vi "PCO_RecorderSaveOverlay_B8.vi"(0 "pImgBufR":u8[][](array[numeric])=array1x4097[4097 elements], 1 "pImgBufG":u8[][](array[numeric])=array1x4097[4097 elements], 2 "pImgBufB":u8[][](array[numeric])=array1x4097[4097 elements], 3 "wWidth":u16, 4 "wHeight":u16, 5 "error in (no error)":errorcluster {"code" format="%x"}, 8 "PCO_METADATA_STRUCT":T1, 9 "szFilePath":path, 11 "bOverwrite":bool) -> (14 "ErrorMessage":i32 format="%x", 19 "error out":errorcluster {"code" format="%x"})   [LabVIEW 2019, in "Recorder.lvlib"]
doc: "int WINAPI PCO_RecorderSaveOverlay(void* pImgBufR, void* pImgBufG, void* pImgBufB, WORD wWidth, WORD wHeight, const char* cFileType, const char* szFilePath, bool bOverwrite, PCO_METADATA_STRUCT* strMetadata);"
uses:
  Recorder.lvlib
  pco.sdk/Structures/Structures.lvlib
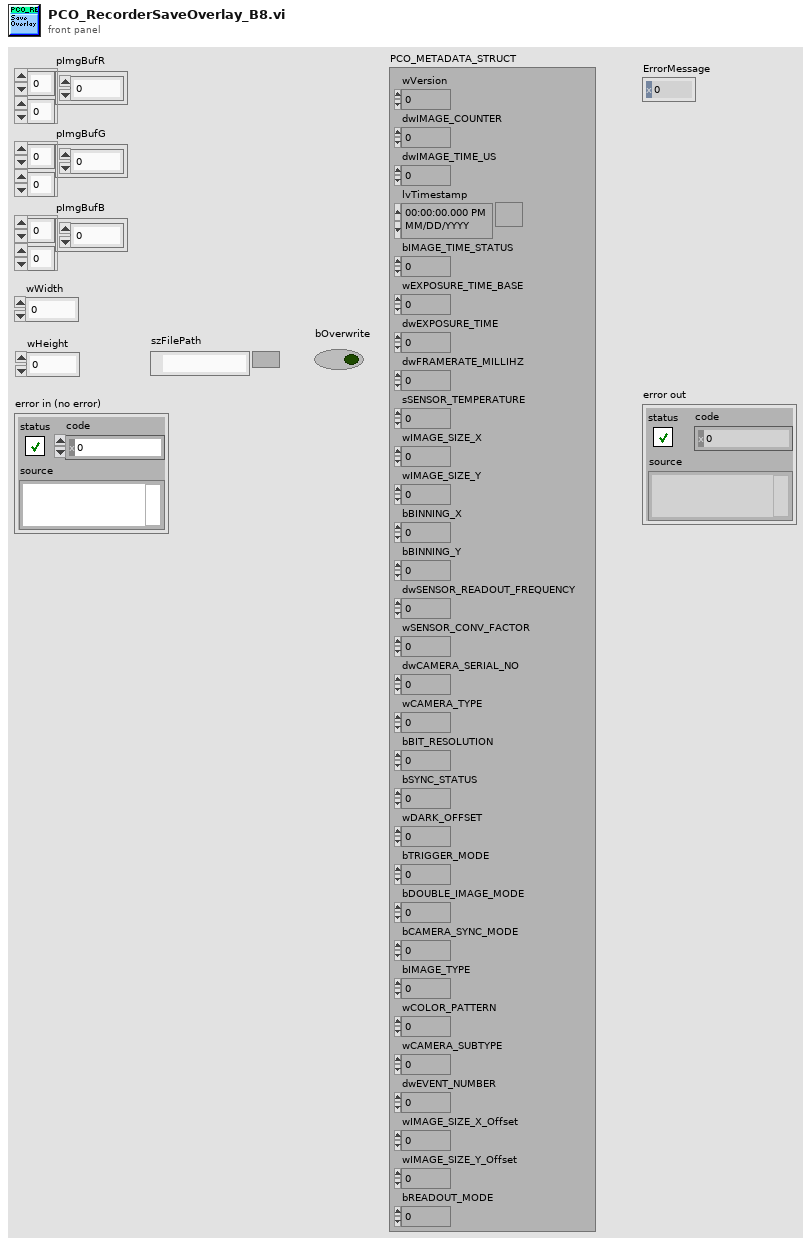
[diagram p1: front panel]
types:
  T1 = cluster{"wVersion":u16, "dwIMAGE_COUNTER":u32, "dwIMAGE_TIME_US":u32, "lvTimestamp":timestamp, "bIMAGE_TIME_STATUS":u8, "wEXPOSURE_TIME_BASE":u16, "dwEXPOSURE_TIME":u32, "dwFRAMERATE_MILLIHZ":u32, "sSENSOR_TEMPERATURE":i16, "wIMAGE_SIZE_X":u16, "wIMAGE_SIZE_Y":u16, "bBINNING_X":u8, "bBINNING_Y":u8, "dwSENSOR_READOUT_FREQUENCY":u32, "wSENSOR_CONV_FACTOR":u16, "dwCAMERA_SERIAL_NO":u32, "wCAMERA_TYPE":u16, "bBIT_RESOLUTION":u8, "bSYNC_STATUS":u8, "wDARK_OFFSET":u16, "bTRIGGER_MODE":u8, "bDOUBLE_IMAGE_MODE":u8, "bCAMERA_SYNC_MODE":u8, "bIMAGE_TYPE":u8, "wCOLOR_PATTERN":u16, "wCAMERA_SUBTYPE":u16, "dwEVENT_NUMBER":u32, "wIMAGE_SIZE_X_Offset":u16, "wIMAGE_SIZE_Y_Offset":u16, "bREADOUT_MODE":u8}
  T2 = typedef "LVDateTimeRec.ctl" = cluster{"fractional second":dbl, "second":i32, "minute":i32, "hour":i32, "day of month":i32, "month":i32, "year":i32, "day of week":i32, "day of year":i32, "DST":i32}
  T3 = cluster{"wSize":u16, "wVersion":u16, "bIMAGE_COUNTER_BCD":cluster{u8, u8, u8, u8}, "bIMAGE_TIME_US_BCD":cluster{u8, u8, u8}, "bIMAGE_TIME_SEC_BCD":u8, "bIMAGE_TIME_MIN_BCD":u8, "bIMAGE_TIME_HOUR_BCD":u8, "bIMAGE_TIME_DAY_BCD":u8, "bIMAGE_TIME_MON_BCD":u8, "bIMAGE_TIME_YEAR_BCD":u8, "bIMAGE_TIME_STATUS":u8, "wEXPOSURE_TIME_BASE":u16, "dwEXPOSURE_TIME":u32, "dwFRAMERATE_MILLIHZ":u32, "sSENSOR_TEMPERATURE":i16, "wIMAGE_SIZE_X":u16, "wIMAGE_SIZE_Y":u16, "bBINNING_X":u8, "bBINNING_Y":u8, "dwSENSOR_READOUT_FREQUENCY":u32, "wSENSOR_CONV_FACTOR":u16, "dwCAMERA_SERIAL_NO":u32, "wCAMERA_TYPE":u16, "bBIT_RESOLUTION":u8, "bSYNC_STATUS":u8, "wDARK_OFFSET":u16, "bTRIGGER_MODE":u8, "bDOUBLE_IMAGE_MODE":u8, "bCAMERA_SYNC_MODE":u8, "bIMAGE_TYPE":u8, "wCOLOR_PATTERN":u16, "wCAMERA_SUBTYPE":u16, "dwEVENT_NUMBER":u32, "wIMAGE_SIZE_X_Offset":u16, "wIMAGE_SIZE_Y_Offset":u16, "bREADOUT_MODE":u8}
  T4 = enum16{"big-endian, network order", "native, host order", "little-endian"}
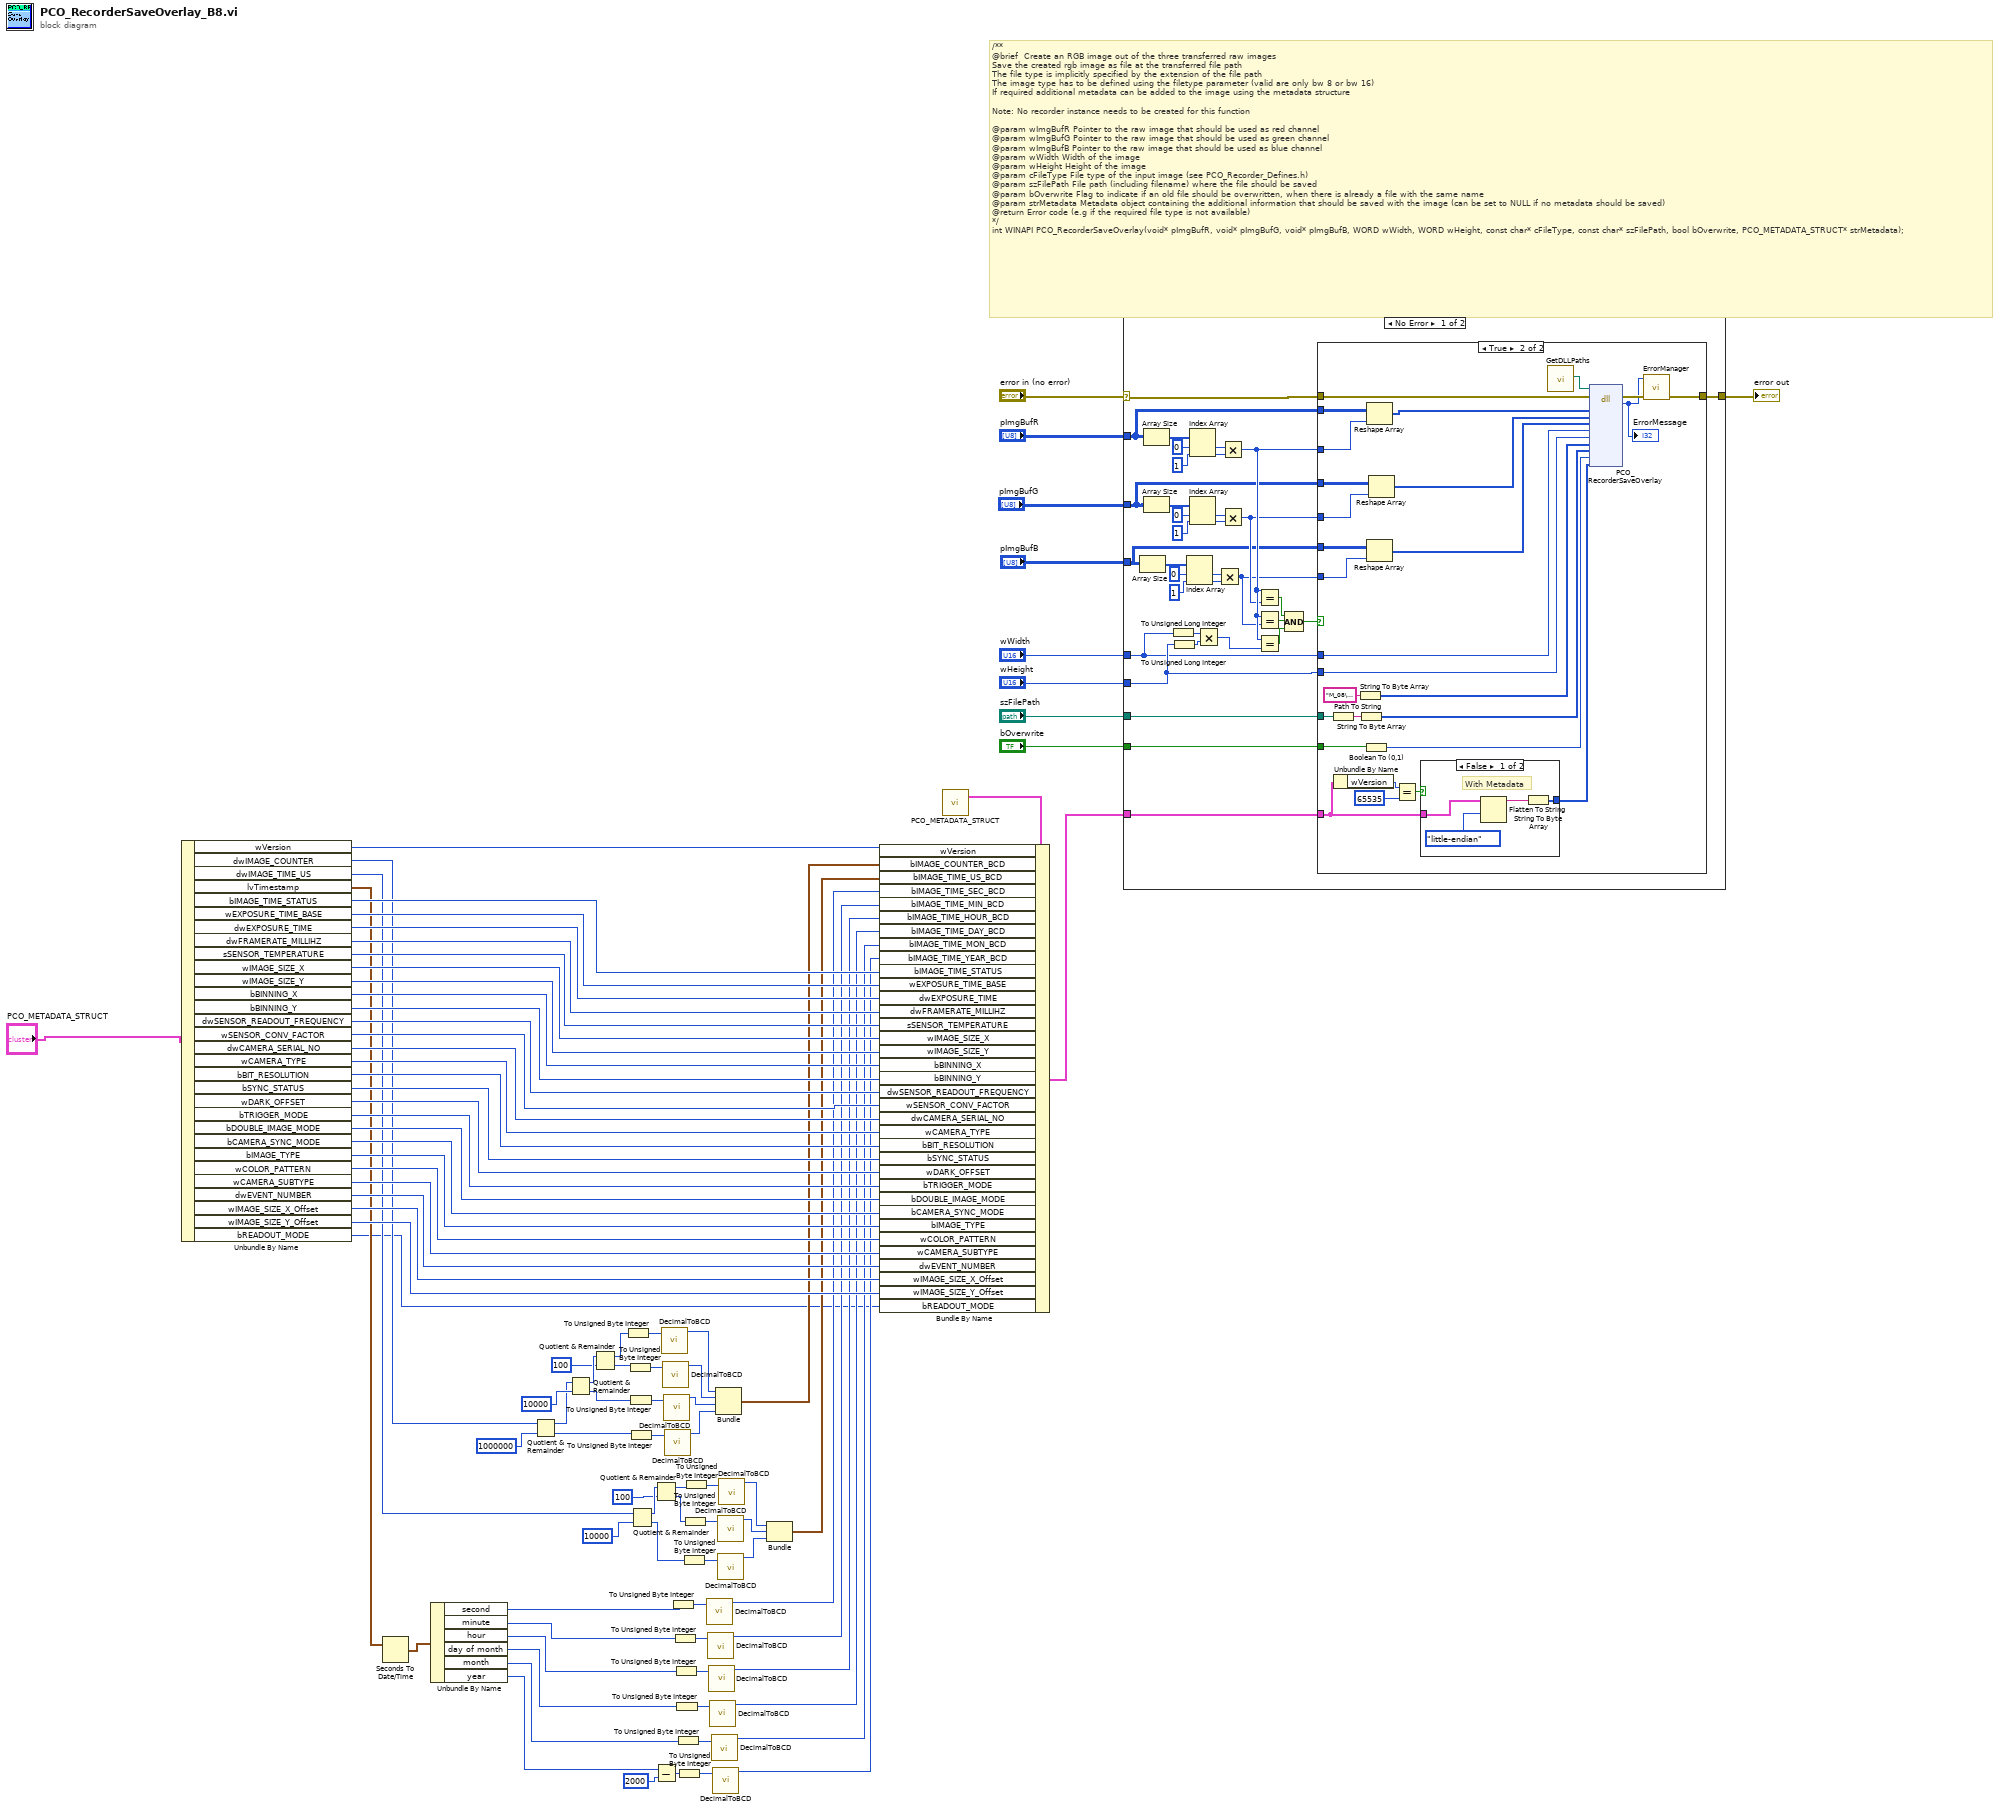
[diagram p0: block diagram]
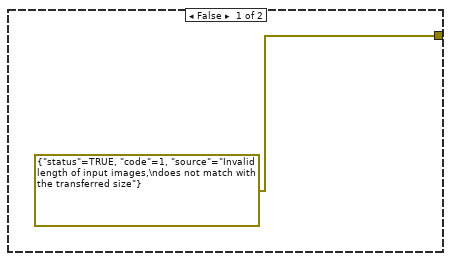
[diagram p2: hidden frame]
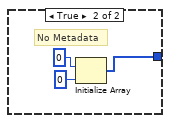
[diagram p3: hidden frame]
diagram:
  # "/**\n@brief  Create an RGB image out of the three transferred raw images\nSave the created rgb image as file at the transferred file path\nThe file type is implicitly specified by the extension of the file path\nThe image type has to be defined using the filetype parameter (valid are only bw 8 or bw 16)\nIf required additional metadata can be added to the image using the metadata structure\n\nNote: No recorder instance needs to be created for this function\n\n@param wImgBufR Pointer to the raw image that should be used as red channel\n@param wImgBufG Pointer to the raw image that should be used as green channel\n@param wImgBufB Pointer to the raw image that should be used as blue channel\n@param wWidth Width of the image\n@param wHeight Height of the image\n@param cFileType File type of the input image (see PCO_Recorder_Defines.h)\n@param szFilePath File path (including filename) where the file should be saved\n@param bOverwrite Flag to indicate if an old file should be overwritten, when there is already a file with the same name\n@param strMetadata Metadata object containing the additional information that should be saved with the image (can be set to NULL if no metadata should be saved)\n@return Error code (e.g if the required file type is not available)\n*/\nint WINAPI PCO_RecorderSaveOverlay(void* pImgBufR, void* pImgBufG, void* pImgBufB, WORD wWidth, WORD wHeight, const char* cFileType, const char* szFilePath, bool bOverwrite, PCO_METADATA_STRUCT* strMetadata);"
  n1 = Unbundle By Name("PCO_METADATA_STRUCT") -> ("wVersion"=w84:u16, "dwIMAGE_COUNTER"=w18:u32, "dwIMAGE_TIME_US"=w23:u32, "lvTimestamp"=w58:timestamp, "bIMAGE_TIME_STATUS"=w72:u8, "wEXPOSURE_TIME_BASE"=w59:u16, "dwEXPOSURE_TIME"=w60:u32, "dwFRAMERATE_MILLIHZ"=w61:u32, "sSENSOR_TEMPERATURE"=w62:i16, "wIMAGE_SIZE_X"=w63:u16, "wIMAGE_SIZE_Y"=w64:u16, "bBINNING_X"=w65:u8, "bBINNING_Y"=w66:u8, "dwSENSOR_READOUT_FREQUENCY"=w67:u32, "wSENSOR_CONV_FACTOR"=w68:u16, "dwCAMERA_SERIAL_NO"=w69:u32, "wCAMERA_TYPE"=w70:u16, "bBIT_RESOLUTION"=w71:u8, "bSYNC_STATUS"=w73:u8, "wDARK_OFFSET"=w74:u16, "bTRIGGER_MODE"=w75:u8, "bDOUBLE_IMAGE_MODE"=w76:u8, "bCAMERA_SYNC_MODE"=w77:u8, "bIMAGE_TYPE"=w78:u8, "wCOLOR_PATTERN"=w79:u16, "wCAMERA_SUBTYPE"=w80:u16, "dwEVENT_NUMBER"=w81:u32, "wIMAGE_SIZE_X_Offset"=w82:u16, "wIMAGE_SIZE_Y_Offset"=w83:u16, "bREADOUT_MODE"=w1:u8)
  n2 = Seconds To Date/Time(time stamp (now)=w58) -> (date time rec=w57:T2)  [unwired: 1 in]
  n3 = Unbundle By Name(w57) -> ("second"=w56:i32, "minute"=w53:i32, "hour"=w48:i32, "day of month"=w47:i32, "month"=w46:i32, "year"=w43:i32)
  n4 = Quotient & Remainder(x=w18, y=u32 1000000 ("x")) -> (x-y*floor(x/y)=w17:u32, floor(x/y)=w12:u32)
  n5 = Quotient & Remainder(x=w17, y=u32 10000 ("x")) -> (x-y*floor(x/y)=w21:u32, floor(x/y)=w11:u32)
  n6 = Quotient & Remainder(x=w21, y=u32 100 ("x")) -> (x-y*floor(x/y)=w9:u32, floor(x/y)=w10:u32)
  n7 = To Unsigned Byte Integer(number=w9) -> (unsigned 8bit integer=w16:u8)
  n8 = To Unsigned Byte Integer(number=w10) -> (unsigned 8bit integer=w15:u8)
  n9 = To Unsigned Byte Integer(number=w11) -> (unsigned 8bit integer=w14:u8)
  n10 = To Unsigned Byte Integer(number=w12) -> (unsigned 8bit integer=w13:u8)
  n11 = Quotient & Remainder(x=w23, y=u32 10000 ("x")) -> (x-y*floor(x/y)=w35:u32, floor(x/y)=w28:u32)
  n12 = Quotient & Remainder(x=w35, y=u32 100 ("x")) -> (x-y*floor(x/y)=w32:u32, floor(x/y)=w30:u32)
  n13 = Subtract(x=w43, y=2000) -> (x-y=w44:i32)
  n14 = call "DecimalToBCD.vi"("U8"=w16) -> ("BCD"=w8:u8)  [unwired: 10 in]
  n15 = call "DecimalToBCD.vi"("U8"=w15) -> ("BCD"=w7:u8)  [unwired: 10 in]
  n16 = call "DecimalToBCD.vi"("U8"=w14) -> ("BCD"=w6:u8)  [unwired: 10 in]
  n17 = call "DecimalToBCD.vi"("U8"=w13) -> ("BCD"=w5:u8)  [unwired: 10 in]
  n18 = To Unsigned Byte Integer(number=w56) -> (unsigned 8bit integer=w55:u8)
  n19 = To Unsigned Byte Integer(number=w53) -> (unsigned 8bit integer=w54:u8)
  n20 = To Unsigned Byte Integer(number=w48) -> (unsigned 8bit integer=w52:u8)
  n21 = To Unsigned Byte Integer(number=w47) -> (unsigned 8bit integer=w49:u8)
  n22 = To Unsigned Byte Integer(number=w46) -> (unsigned 8bit integer=w50:u8)
  n23 = To Unsigned Byte Integer(number=w44) -> (unsigned 8bit integer=w51:u8)
  n24 = To Unsigned Byte Integer(number=w28) -> (unsigned 8bit integer=w29:u8)
  n25 = To Unsigned Byte Integer(number=w30) -> (unsigned 8bit integer=w31:u8)
  n26 = To Unsigned Byte Integer(number=w32) -> (unsigned 8bit integer=w33:u8)
  n27 = call "DecimalToBCD.vi"("U8"=w55) -> ("BCD"=w37:u8)  [unwired: 10 in]
  n28 = call "DecimalToBCD.vi"("U8"=w54) -> ("BCD"=w38:u8)  [unwired: 10 in]
  n29 = call "DecimalToBCD.vi"("U8"=w52) -> ("BCD"=w39:u8)  [unwired: 10 in]
  n30 = call "DecimalToBCD.vi"("U8"=w49) -> ("BCD"=w40:u8)  [unwired: 10 in]
  n31 = call "DecimalToBCD.vi"("U8"=w50) -> ("BCD"=w41:u8)  [unwired: 10 in]
  n32 = call "DecimalToBCD.vi"("U8"=w51) -> ("BCD"=w42:u8)  [unwired: 10 in]
  n33 = Bundle("BCD"=w8, "BCD"=w7, "BCD"=w6, "BCD"=w5) -> (w4:cluster{"BCD":u8, "BCD":u8, "BCD":u8, "BCD":u8})  [unwired: 1 in]
  n34 = call "DecimalToBCD.vi"("U8"=w29) -> ("BCD"=w25:u8)  [unwired: 10 in]
  n35 = call "DecimalToBCD.vi"("U8"=w31) -> ("BCD"=w26:u8)  [unwired: 10 in]
  n36 = call "DecimalToBCD.vi"("U8"=w33) -> ("BCD"=w27:u8)  [unwired: 10 in]
  n37 = Bundle("BCD"=w27, "BCD"=w26, "BCD"=w25) -> (w24:cluster{"BCD":u8, "BCD":u8, "BCD":u8})  [unwired: 1 in]
  n38 = call "PCO_METADATA_STRUCT.vi"() -> ("PCO_METADATA_STRUCT_Raw"=w85:T3)  [unwired: 4 in, 3 out]
  n39 = Bundle By Name(cluster=w85, "wVersion"=w84, "bIMAGE_COUNTER_BCD"=w4, "bIMAGE_TIME_US_BCD"=w24, "bIMAGE_TIME_SEC_BCD"=w37, "bIMAGE_TIME_MIN_BCD"=w38, "bIMAGE_TIME_HOUR_BCD"=w39, "bIMAGE_TIME_DAY_BCD"=w40, "bIMAGE_TIME_MON_BCD"=w41, "bIMAGE_TIME_YEAR_BCD"=w42, "bIMAGE_TIME_STATUS"=w72, "wEXPOSURE_TIME_BASE"=w59, "dwEXPOSURE_TIME"=w60, "dwFRAMERATE_MILLIHZ"=w61, "sSENSOR_TEMPERATURE"=w62, "wIMAGE_SIZE_X"=w63, "wIMAGE_SIZE_Y"=w64, "bBINNING_X"=w65, "bBINNING_Y"=w66, "dwSENSOR_READOUT_FREQUENCY"=w67, "wSENSOR_CONV_FACTOR"=w68, "dwCAMERA_SERIAL_NO"=w69, "wCAMERA_TYPE"=w70, "bBIT_RESOLUTION"=w71, "bSYNC_STATUS"=w73, "wDARK_OFFSET"=w74, "bTRIGGER_MODE"=w75, "bDOUBLE_IMAGE_MODE"=w76, "bCAMERA_SYNC_MODE"=w77, "bIMAGE_TYPE"=w78, "wCOLOR_PATTERN"=w79, "wCAMERA_SUBTYPE"=w80, "dwEVENT_NUMBER"=w81, "wIMAGE_SIZE_X_Offset"=w82, "wIMAGE_SIZE_Y_Offset"=w83, "bREADOUT_MODE"=w1) -> (w3:T3)
  n40 = case shown="No Error" "error in (no error)" {
    selector: "error in (no error)" -> [w129 w166]
    tunnel: "pImgBufR" -> [w119 _]
    tunnel: "pImgBufG" -> [w107 _]
    tunnel: "pImgBufB" -> [w100 _]
    tunnel: "wWidth" -> [w95 _]
    tunnel: "wHeight" -> [w96 _]
    tunnel: "szFilePath" -> [w120 _]
    tunnel: [w128 w166] -> w87
    tunnel: "bOverwrite" -> [w127 _]
    tunnel: w3 -> [w121 _]
    frame No Error {
      n41 = Array Size(array=w100) -> (size(s)=w105:i32[])
      n42 = Array Size(array=w119) -> (size(s)=w118:i32[])
      n43 = Array Size(array=w107) -> (size(s)=w108:i32[])
      n44 = To Unsigned Long Integer(number=w95) -> (unsigned 32bit integer=w98:u32)
      n45 = To Unsigned Long Integer(number=w96) -> (unsigned 32bit integer=w97:u32)
      n46 = Index Array(array=w105, index #1=0 ("index"), index #2=1 ("index")) -> (element #1=w101:i32, element #2=w102:i32)
      n47 = Index Array(array=w118, index #1=0 ("index"), index #2=1 ("index")) -> (element #1=w114:i32, element #2=w115:i32)
      n48 = Index Array(array=w108, index #1=0 ("index"), index #2=1 ("index")) -> (element #1=w112:i32, element #2=w111:i32)
      n49 = Multiply(x=w98, y=w97) -> (x*y=w126:u32)
      n50 = Multiply(x=w101, y=w102) -> (x*y=w99:i32)
      n51 = Multiply(x=w114, y=w115) -> (x*y=w113:i32)
      n52 = Multiply(x=w112, y=w111) -> (x*y=w106:i32)
      n53 = Equal?(x=w113, y=w106) -> (x = y?=w125:bool)
      n54 = Equal?(x=w113, y=w99) -> (x = y?=w124:bool)
      n55 = Equal?(x=w113, y=w126) -> (x = y?=w123:bool)
      n56 = Compound Arithmetic op=AND(w125, w124, w123) -> (w122:bool)
      n57 = case shown="True" w122 {
        tunnel: w129 -> [_ w158]
        tunnel: [errorcluster {"status"=TRUE, "code"=1, "source"="Invalid length of input images,\ndoes not match with the transferred size"} ("error out") w155] -> w128
        tunnel: w127 -> [_ w153]
        tunnel: w121 -> [_ w148]
        tunnel: w120 -> [_ w146]
        tunnel: w119 -> [_ w139]
        tunnel: w107 -> [_ w138]
        tunnel: w100 -> [_ w137]
        tunnel: w95 -> [_ w142]
        tunnel: w96 -> [_ w141]
        tunnel: w113 -> [_ w134]
        tunnel: w106 -> [_ w135]
        tunnel: w99 -> [_ w136]
        frame False {
        }
        frame True {
          n58 = Path To String(path=w146) -> (string=w147:string)
          n59 = Unbundle By Name(w148) -> ("wVersion"=w151:u16)
          n60 = String To Byte Array(string="M_08\u0000") -> (unsigned byte array=w143:u8[])
          n61 = String To Byte Array(string=w147) -> (unsigned byte array=w144:u8[])
          n62 = Boolean To (0,1)(Boolean=w153) -> (0, 1=w152:i16)
          n63 = Reshape Array(w139, w134) -> (w133:u8[])
          n64 = Reshape Array(w137, w136) -> (w131:u8[])
          n65 = Reshape Array(w138, w135) -> (w132:u8[])
          n66 = Equal?(x=w151, y=u16 65535) -> (x = y?=w149:bool)
          n67 = case shown="False" w149 {
            tunnel: [w160 w163] -> w140
            tunnel: w148 -> [w161 _]
            frame False {
              # "With Metadata"
              n68 = Flatten To String(anything=w161, byte order (0:big-endian, network order)=T4."little-endian" ("Byte-Reihenfolge (0:Big-Endian, Netzwerkreihenfolge)")) -> (data string=w162:string)  [unwired: 2 in, 2 out]
              n69 = String To Byte Array(string=w162) -> (unsigned byte array=w160:u8[])
            }
            frame True {
              # "No Metadata"
              n70 = Initialize Array(u8 0, 0 ("dimension size")) -> (w163:u8[])
            }
          }
          n71 = call "GetDLLPaths.vi"() -> ("PCO_Recorder_Path"=w157:path)  [unwired: 8 in, 3 out]
          n72 = dll-call lib="?" fn="PCO_RecorderSaveOverlay"(path in=w157, error in=w158, "pImgBufR"=w133, "pImgBufG"=w132, "pImgBufB"=w131, "wWidth"=w142, "wHeight"=w141, "cFileType"=w143, "szFilePath"=w144, "bOverwrite"=w152, "strMetadata"=w140) -> (error out=w156:errorcluster, "return type"=w154:i32)  [unwired: 10 in, 1 out]
          "ErrorMessage" <- w154
          n73 = call "ErrorManager.vi"("error in (no error)"=w156, "error code"=w154) -> ("error out"=w155:errorcluster)  [unwired: 2 in, 1 out]
        }
      }
    }
    frame Error {
    }
  }
  "error out" <- w87
